vi "Test_TDelay_bin.vi"() -> ()   [LabVIEW 2022 SP3]
panel:
  in  "stop":bool
  out "Waveform Chart":i16[][](graph)
  in  "delay":i32=1
  in  "input":bool
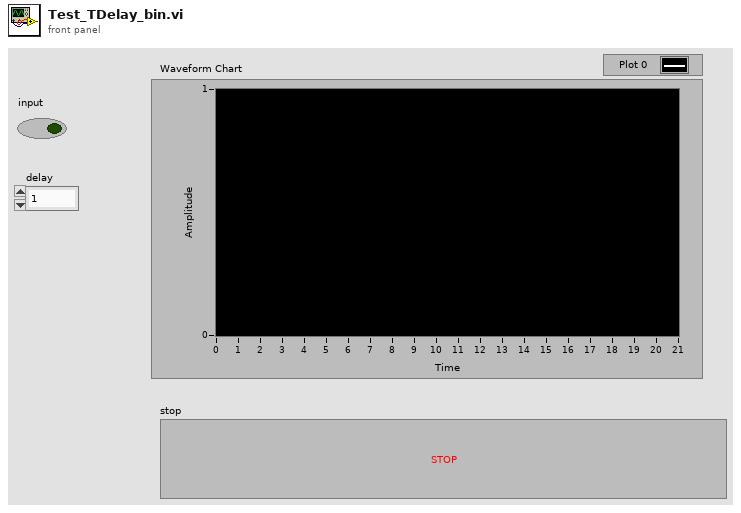
[diagram p1: front panel]
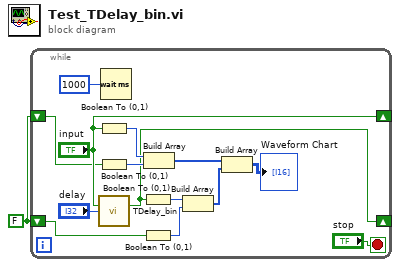
[diagram p0: block diagram]
diagram:
  w1 = FALSE ("input")
  n1 = while {
    shift-right: ["input"] -> _
    shift-left: w1 -> [w8]
    shift-right: [w6] -> _
    shift-left: w1 -> [w4]
    stop <- "stop" stop-if-true
    n2 = Boolean To (0,1)(Boolean="input") -> (0, 1=w10:i16)
    n3 = Boolean To (0,1)(Boolean=w8) -> (0, 1=w9:i16)
    n4 = call "TDelay_bin.vi"("Boolean"="input", "delay"="delay") -> ("output"=w6:bool)  [unwired: 12 in, 1 out]
    n5 = Wait (ms)(milliseconds to wait=u32 1000) -> ()  [unwired: 1 out]
    n6 = Boolean To (0,1)(Boolean=w6) -> (0, 1=w5:i16)
    n7 = Boolean To (0,1)(Boolean=w4) -> (0, 1=w3:i16)
    n8 = Build Array(w10, w9) -> (w7:i16[])
    n9 = Build Array(w5, w3) -> (w2:i16[])
    n10 = Build Array(w7, w2) -> (→"Waveform Chart":i16[][])
  }
